vi "Subvi sample and hold U8.vi"(6 "Reset":bool, 8 "Refresh":bool, 9 "Input":u8) -> (1 "Output":u8)   [LabVIEW 2017]
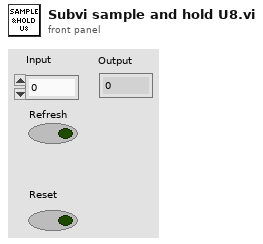
[diagram p1: front panel]
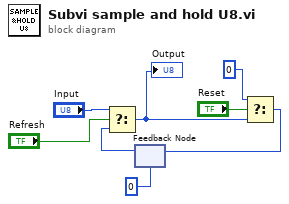
[diagram p0: block diagram]
diagram:
  n1 = feedback #1(u8 0) -> (w3:u8)
  n2 = Select(t="Input", s="Refresh", f=w3) -> (s? t:f=w4:u8)
  "Output" <- w4
  n3 = Select(t=u8 0, s="Reset", f=w4) -> (s? t:f=w7:u8)
  n4 = feedback-in #1(w7) -> ()
